vi "write_active_channels.vi"(8 "error in (no error)":errorcluster, 10 "active_channels":u32[](array[numeric])=[0, 1], 11 "tt20 in":refnum<class "tt20.lvclass">) -> (0 "error out":errorcluster, 3 "tt20 out":refnum<class "tt20.lvclass">)   [LabVIEW 2015, in "tt20.lvclass"]
uses:
  tt20.lvclass
  tt20.lvclass/tt20.ctl
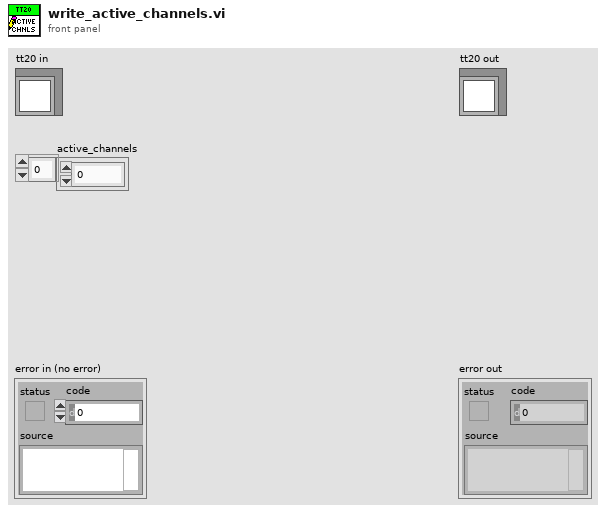
[diagram p1: front panel]
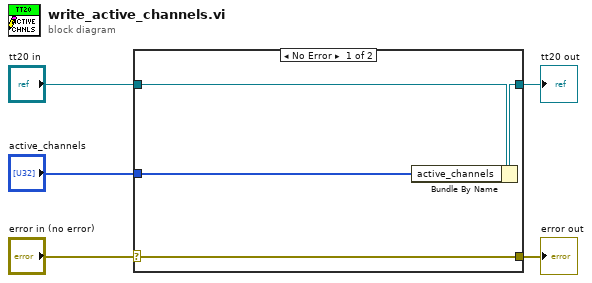
[diagram p0: block diagram]
diagram:
  n1 = case shown="No Error" "error in (no error)" {
    selector: "error in (no error)" -> [w9 w10]
    tunnel: [w9 w10] -> w4
    tunnel: [w7 w11] -> w2
    tunnel: "tt20 in" -> [w8 w11]
    tunnel: "active_channels" -> [w6 _]
    frame No Error {
      n2 = Bundle By Name(cluster=w8, "active_channels"=w6) -> (w7:refnum<class "tt20.lvclass">)
    }
    frame Error {
    }
  }
  "error out" <- w4
  "tt20 out" <- w2
